vi "GetPose.vi"(11 "QTM ID":i32) -> (3 "Pose":sgl[](array[numeric]))   [LabVIEW 2013]
uses:
  <userlib>/QLC/QLC.lvlib
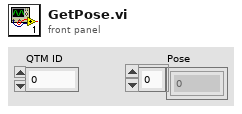
[diagram p1: front panel]
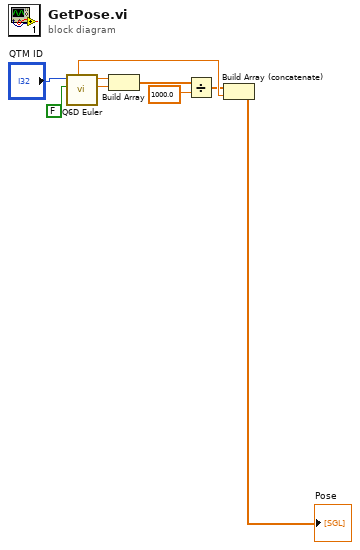
[diagram p0: block diagram]
diagram:
  n1 = call <userlib>:"Q6D Euler.vi"("residual"=FALSE, "no"="QTM ID") -> ("y"=w7:sgl, "x"=w6:sgl, "yaw"=w8:sgl)  [unwired: 3 in, 4 out]
  n2 = Build Array(w6, w7) -> (w3:sgl[])
  n3 = Divide(x=w3, y=sgl 1000.0) -> (x/y=w5:sgl[])
  n4 = Build Array (concatenate)(w5, w8) -> (→"Pose":sgl[])
